vi "Range.vi"(7 "Set? (F:Read)":bool, 8 "Error In":errorcluster, 9 "Range (1 SCCM)":T1(ring), 10 "Channel (0)":i32, 11 "VISA resource name":refnum<visa-resource-name>) -> (0 "Error Out":errorcluster, 1 "Range out":T1(ring), 3 "dup VISA resource name":refnum<visa-resource-name>)   [LabVIEW 2011, in "MGC647C.lvlib"]
doc: "Read/Set range of a channel."
uses:
  <instrlib>/MGC647C/MGC647C.lvlib
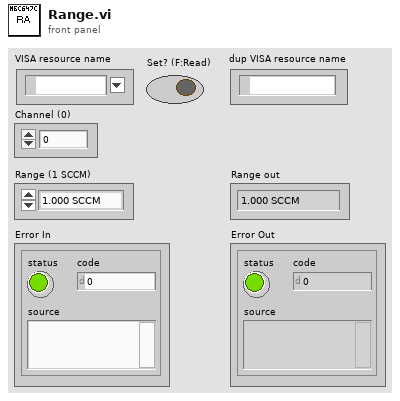
[diagram p1: front panel]
types:
  T1 = enum16{"1.000 SCCM", "2.000 SCCM", "5.000 SCCM", "10.00 SCCM", "20.00 SCCM", "50.00 SCCM", "100.0 SCCM", "200.0 SCCM", "500.0 SCCM", "1.000 SLM", "2.000 SLM", "5.000 SLM", "10.00 SLM", "20.00 SLM", "50.00 SLM", "100.0 SLM", "200.0 SLM", "400.0 SLM", "500.0 SLM", "1.000 SCMM", "1.000 SCFH", "2.000 SCFH", "5.000 SCFH", "10.00 SCFH", "20.00 SCFH", "50.00 SCFH", "100.0 SCFH", "200.0 SCFH", "500.0 SCFH", "1.000 SCFM", "2.000 SCFM", "5.000 SCFM", "10.00 SCFM", "20.00 SCFM", "50.00 SCFM", "100.0 SCFM", "200.0 SCFM", "500.0 SCFM", "30.00 SLM", "300.0 SLM"}
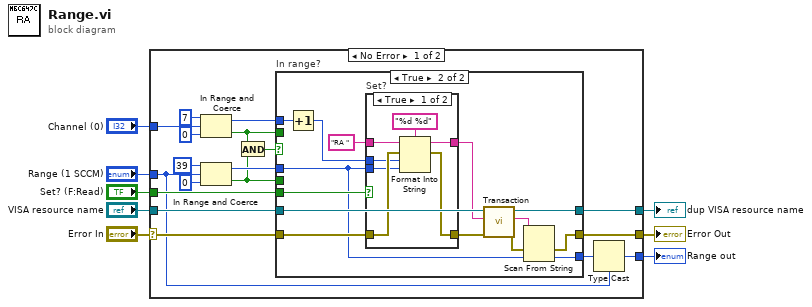
[diagram p0: block diagram]
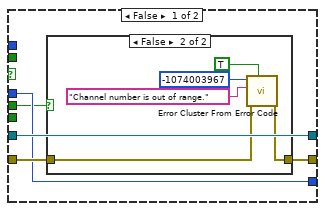
[diagram p2: hidden frame]
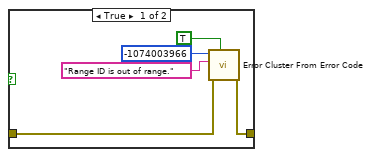
[diagram p3: hidden frame]
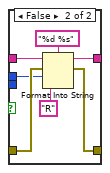
[diagram p4: hidden frame]
diagram:
  n1 = case shown="No Error" "Error In" {
    selector: "Error In" -> [w19 w71]
    tunnel: "VISA resource name" -> [w26 w70]
    tunnel: [w25 w70] -> w7
    tunnel: [w24 w71] -> w6
    tunnel: "Set? (F:Read)" -> [w23 _]
    tunnel: "Range (1 SCCM)" -> [w9 w72]
    tunnel: [w10 w72] -> w2
    tunnel: "Channel (0)" -> [w16 _]
    frame No Error {
      n2 = In Range and Coerce(upper limit=7, x=w16, lower limit=0) -> (coerced(x)=w15:i32, In Range?=w13:bool)
      n3 = In Range and Coerce(upper limit=u16 39, x=w9, lower limit=u16 0) -> (coerced(x)=w22:u16, In Range?=w12:bool)
      n4 = And(x=w13, y=w12) -> (x .and. y?=w14:bool)
      n5 = case "In range?" shown="True" w14 {
        tunnel: w26 -> [w29 w55]
        tunnel: [w29 w54] -> w25
        tunnel: [w30 w49] -> w24
        tunnel: w23 -> [_ w44]
        tunnel: w22 -> [w28 w43]
        tunnel: w19 -> [w31 w53]
        tunnel: [w28 w42] -> w11
        tunnel: w15 -> [_ w48]
        tunnel: w13 -> [_ _]
        tunnel: w12 -> [w27 _]
        frame False {
          n6 = case shown="False" w27 {
            tunnel: w31 -> [w36 w41]
            tunnel: [w35 w40] -> w30
            frame True {
              n7 = call <vilib>:"Error Cluster From Error Code.vi"("show call chain? (False)"=TRUE, "error in (no error)"=w36, "error message (\"\")"="Range ID is out of range." ("error message (\"\")"), "error code (0)"=-1074003966) -> ("error out"=w35:errorcluster)  [unwired: 5 in]
            }
            frame False {
              n8 = call <vilib>:"Error Cluster From Error Code.vi"("show call chain? (False)"=TRUE, "error in (no error)"=w41, "error message (\"\")"="Channel number is out of range." ("error message (\"\")"), "error code (0)"=-1074003967) -> ("error out"=w40:errorcluster)  [unwired: 5 in]
            }
          }
        }
        frame True {
          n9 = Increment(x=w48) -> (x+1=w47:i32)
          n10 = case "Set?" shown="True" w44 {
            tunnel: w53 -> [w62 w69]
            tunnel: [w61 w68] -> w52
            tunnel: w47 -> [w60 w67]
            tunnel: w43 -> [w59 _]
            tunnel: "RA " ("string (\"\")") -> [w58 w66]
            tunnel: [w57 w65] -> w45
            frame True {
              n11 = Format Into String(format string="%d %d", initial string=w58, error in=w62, w60, w59) -> (resulting string=w57:string, error out=w61:errorcluster)
            }
            frame False {
              n12 = Format Into String(format string="%d %s", initial string=w66, error in=w69, w67, "R") -> (resulting string=w65:string, error out=w68:errorcluster)
            }
          }
          n13 = call <instrlib>:"Transaction.vi"("Error In"=w52, "Command"=w45, "VISA resource name"=w55) -> ("Error Out"=w50:errorcluster, "Response"=w51:string, "dup VISA resource name"=w54:refnum<visa-resource-name>)  [unwired: 6 in]
          n14 = Scan From String(input string=w51, error in=w50, default 1=w43) -> (error out=w49:errorcluster, output 1=w42:u16)  [unwired: 2 in, 2 out]
        }
      }
      n15 = Type Cast(type=w9, x=w11) -> (*(type *) &x=w10:T1)
    }
    frame Error {
    }
  }
  "dup VISA resource name" <- w7
  "Error Out" <- w6
  "Range out" <- w2
